vi "XXXXXXXXXX.vi"() -> ()   [LabVIEW 2009]
panel:
  out "In Range?":bool[](array[boolean])
  out "Numeric 2":dbl
  out "Numeric":dbl
  out "Array":bool[][][](array[boolean])
  out "x = y?":bool
  in  "LOW":dbl[][](array[numeric])=[[0.021, 0.021, 0.021, 0.5, 0.5, 0.5, 0.11, 0.11, 0.11], [0.11, 0.11, 0.11, 0.189, 0.189, 0.189, 0.27, 0.27, 0.27], [0.27, 0.27, 0.27, 0.421, 0.421, 0.421, 0.551, 0.551, 0.551]]
  in  "HIGH":dbl[][](array[numeric])=[[0.15, 0.15, 0.15, 0.2, 0.2, 0.2, 0.242, 0.242, 0.242], [0.242, 0.242, 0.242, 0.331, 0.331, 0.331, 0.425, 0.425, 0.425], [0.425, 0.425, 0.425, 0.6, 0.6, 0.6, 0.774, 0.774, 0.774]]
  out "Volt LLTH Corregido":dbl[](array[numeric])
  in  "Salida A rectificada":dbl[][][](array[numeric])
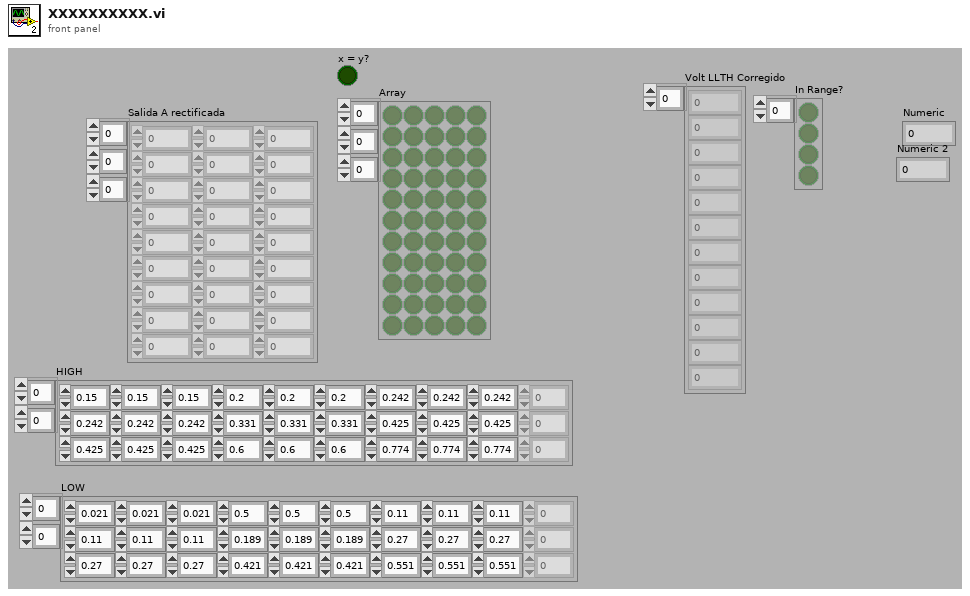
[diagram p1: front panel]
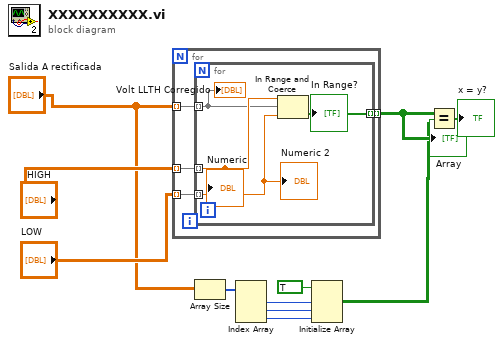
[diagram p0: block diagram]
diagram:
  n1 = for {
    tunnel: "Salida A rectificada" -> [w12] mode=indexing
    tunnel: [w15] -> w6 mode=indexing
    tunnel: "HIGH" -> [w14] mode=indexing
    tunnel: "LOW" -> [w13] mode=indexing
    n2 = for {
      tunnel: w12 -> [w16] mode=indexing
      tunnel: [w19] -> w15 mode=indexing
      tunnel: w14 -> [w18] mode=indexing
      tunnel: w13 -> [w17] mode=indexing
      n3 = In Range and Coerce(upper limit=w18, x=w16, lower limit=w17) -> (In Range?=w19:bool[])  [unwired: 1 out]
      "In Range?" <- w19
      "Volt LLTH Corregido" <- w16
      "Numeric" <- w18
      "Numeric 2" <- w17
    }
  }
  "Array" <- w6
  n4 = Array Size(array="Salida A rectificada") -> (size(s)=w11:i32[])
  n5 = Index Array(array=w11) -> (element #1=w10:i32, element #2=w9:i32, element #3=w8:i32)  [unwired: 3 in]
  n6 = Initialize Array(TRUE, w10, w9, w8) -> (w3:bool[][][])
  n7 = Equal?(x=w6, y=w3) -> (x = y?=→"x = y?":bool)
